vi "Read Standard.vi"(8 "error in (no error)":errorcluster, 11 "Harmonics_Relative_Power in":refnum<class "Harmonics_Relative_Power.lvclass">) -> (0 "error out":errorcluster, 2 "Standard":string, 3 "Harmonics_Relative_Power out":refnum<class "Harmonics_Relative_Power.lvclass">)   [LabVIEW 2018, in "SeqAuto Evaluations.lvlib" / "Harmonics_Relative_Power.lvclass"]
uses:
  Harmonics_Relative_Power.lvclass
  Harmonics_Relative_Power.lvclass/Harmonics_Relative_Power.ctl
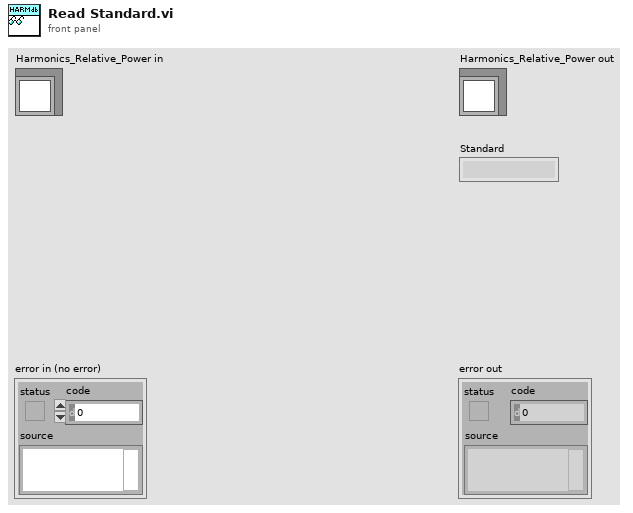
[diagram p1: front panel]
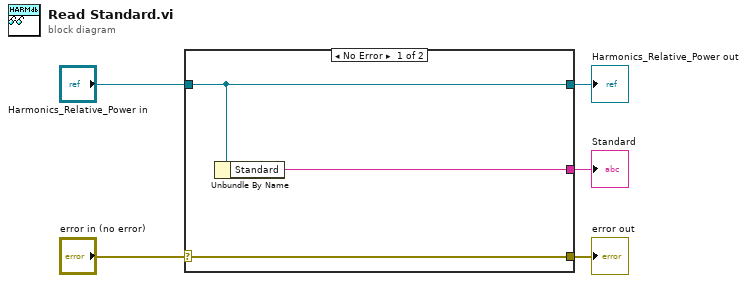
[diagram p0: block diagram]
diagram:
  n1 = case shown="No Error" "error in (no error)" {
    selector: "error in (no error)" -> [w8 w9]
    tunnel: [w8 w9] -> w4
    tunnel: [w7 w10] -> w2
    tunnel: "Harmonics_Relative_Power in" -> [w7 w10]
    tunnel: [w6 _] -> w1
    frame No Error {
      n2 = Unbundle By Name(w7) -> ("Standard"=w6:string)
    }
    frame Error {
    }
  }
  "error out" <- w4
  "Harmonics_Relative_Power out" <- w2
  "Standard" <- w1
